vi "GPOCT_Process.vi"(8 "error in (no error)":errorcluster, 9 "Array in":u16[](array[numeric]), 10 "SizeParam":i32[](array[numeric]), 11 "path in":path) -> (0 "error out":errorcluster, 2 "Array":cdb[](array[numeric]), 3 "path out":path)   [LabVIEW 2016]
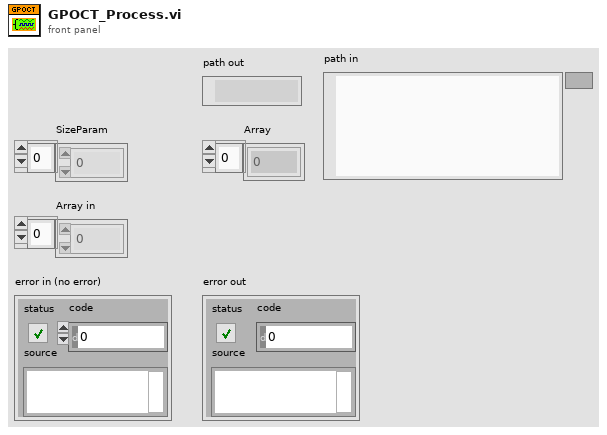
[diagram p1: front panel]
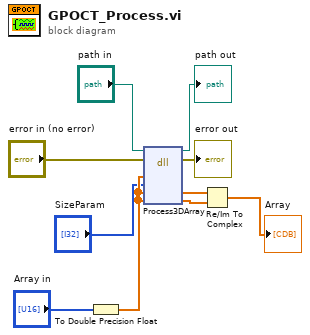
[diagram p0: block diagram]
diagram:
  n1 = To Double Precision Float(number="Array in") -> (double precision float=w7:dbl[])
  n2 = dll-call lib="C:/Users/Mikael/Documents/Visual Studio 2015/Projects/GPOCT/x64/Release/GPOCT.dll" fn="Process3DArray"(path in="path in", error in="error in (no error)", "input"=w7, "size"="SizeParam", "output_real"=w7, "output_imag"=w7) -> (path out=→"path out":path, error out=→"error out":errorcluster, "output_real"=w8:dbl[], "output_imag"=w9:dbl[])  [unwired: 4 in]
  n3 = Re/Im To Complex(1:w9, 2:w8) -> (0:→"Array":cdb[])
